vi "Init Events.vi"(8 "error in (no error)":errorcluster, 11 "Value Editor Base in":refnum<class "Value Editor Base.lvclass">) -> (0 "error out":errorcluster, 3 "Value Editor Base out":refnum<class "Value Editor Base.lvclass">)   [LabVIEW 2020, in "Value Editor Base.lvclass"]
uses:
  Value Editor Base.lvclass
  Update Type Data.ctl
  Type Descriptor.ctl
  Terminal Direction.ctl
  Value Mode.ctl
  Special Terminal.ctl
  Terminal Mode Data.ctl
  Terminal Mode.ctl
  Update Value Data.ctl
  Value Editor Base.lvclass/Value Editor Base.ctl
  FlexBlocks.lvlib
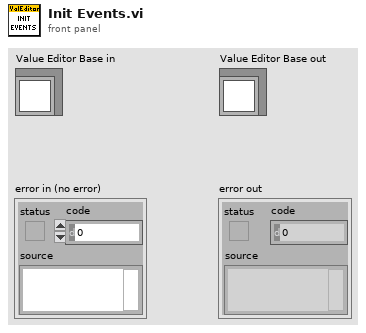
[diagram p1: front panel]
types:
  T1 = typedef "Value Editor Base.lvclass/Update Value Data.ctl" = cluster{"Value":variant}
  T2 = typedef "Value Editor Base.lvclass/Terminal Mode Data.ctl" = cluster{"Terminal Mode":T3}
  T3 = typedef "FlexBlocks.lvlib/Terminal Mode.ctl" = enum16{"Channel", "Config", "Value", "Control Ref"}
  T4 = typedef "Value Editor Base.lvclass/Update Type Data.ctl" = cluster{"Type":T5}
  T5 = typedef "FlexBlocks.lvlib/Type Descriptor.ctl" = cluster{"Name":string, "Direction":T6, "Default":variant, "Min":variant, "Max":variant, "Step":variant, "Value Mode":T7, "Required":bool, "Connpane Index":i32, "Special Terminal":T8, "Color":u32, "Options":string[], "Type String":string, "Sort":i32, "Item Path":path}
  T6 = typedef "FlexBlocks.lvlib/Terminal Direction.ctl" = enum16{"Sink", "Source"}
  T7 = typedef "FlexBlocks.lvlib/Value Mode.ctl" = enum16{"Normal", "Range", "Select"}
  T8 = typedef "FlexBlocks.lvlib/Special Terminal.ctl" = enum16{"None", "Action", "Init", "Tag", "State in", "State out", "Error"}
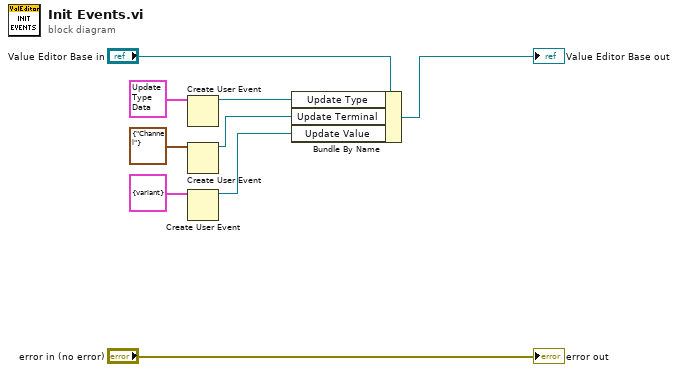
[diagram p0: block diagram]
diagram:
  n1 = Create User Event(user event datatype=T4 {"Type"={"Name"="", "Direction"=enum."Sink", "Default"=variant, "Min"=variant, "Max"=variant, "Step"=variant, "Value Mode"=enum."Normal", "Required"=FALSE, "Connpane Index"=0, "Special Terminal"=enum."None", "Color"=0, "Options"=[], "Type String"="", "Sort"=0, "Item Path"=path ""}} ("Update Type Data")) -> (user event=w5:refnum<user-event>)  [unwired: 1 in, 1 out]
  n2 = Create User Event(user event datatype=T2 {"Terminal Mode"=enum."Channel"} ("Terminal Type Data")) -> (user event=w3:refnum<user-event>)  [unwired: 1 in, 1 out]
  n3 = Create User Event(user event datatype=T1 {"Value"=variant} ("Update Value Data")) -> (user event=w1:refnum<user-event>)  [unwired: 1 in, 1 out]
  n4 = Bundle By Name(cluster="Value Editor Base in", "Update Type"=w5, "Update Terminal"=w3, "Update Value"=w1) -> (→"Value Editor Base out":refnum<class "Value Editor Base.lvclass">)
  "error out" <- "error in (no error)"
